vi "readStopAcq.vi"(8 "error in (no error)":errorcluster, 11 "Acquisition in":refnum<class "Acquisition.lvclass">) -> (0 "error out":errorcluster, 2 "ERROR STOP":bool, 3 "Acquisition out":refnum<class "Acquisition.lvclass">)   [LabVIEW 2014, in "Acquisition.lvclass"]
uses:
  Acquisition.lvclass
  Acquisition.lvclass/Acquisition.ctl
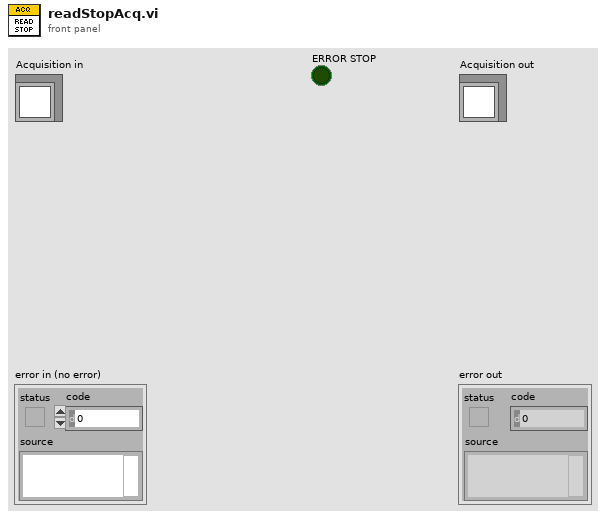
[diagram p1: front panel]
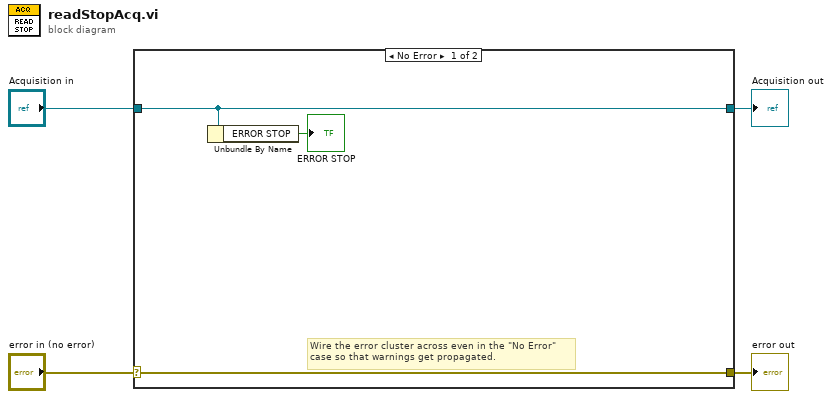
[diagram p0: block diagram]
diagram:
  n1 = case shown="No Error" "error in (no error)" {
    selector: "error in (no error)" -> [w7 w9]
    tunnel: [w7 w9] -> w3
    tunnel: [w6 w8] -> w1
    tunnel: "Acquisition in" -> [w6 w8]
    frame No Error {
      # "Wire the error cluster across even in the \"No Error\"\ncase so that warnings get propagated."
      n2 = Unbundle By Name(w6) -> ("ERROR STOP"=→"ERROR STOP":bool)
    }
    frame Error {
    }
  }
  "error out" <- w3
  "Acquisition out" <- w1
